vi "Read or create tokens.vi"(8 "error in":errorcluster, 10 "default value":string, 11 "key":string) -> (0 "error out":errorcluster, 3 "value":string)   [LabVIEW 2021, in "IconEditorDefaultPlugin.lvlib" / "IconEditorDefaultPlugin.lvclass"]
uses:
  <resource>/plugins/NIIconEditor/UI/Default/IconEditorDefaultPlugin.lvclass
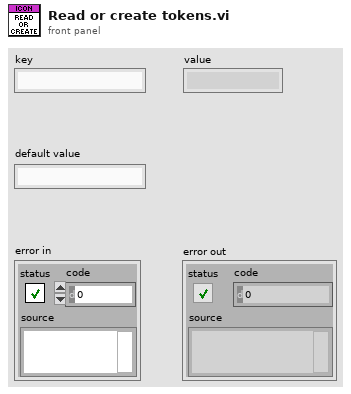
[diagram p1: front panel]
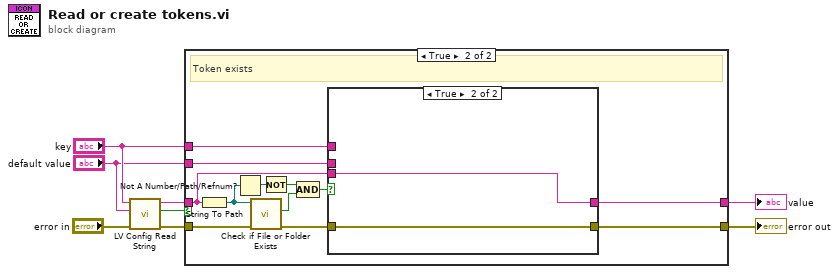
[diagram p0: block diagram]
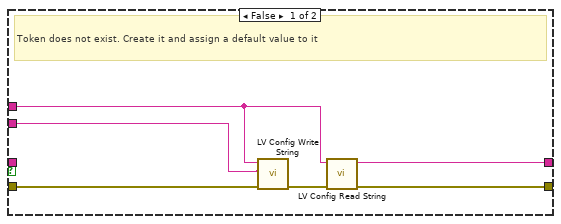
[diagram p2: hidden frame]
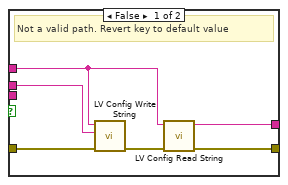
[diagram p3: hidden frame]
diagram:
  n1 = call <resource>:"LV Config Read String.vi"("error in"="error in", "default value"="default value", "key"="key") -> ("error out"=w7:errorcluster, "found?"=w6:bool, "value"=w2:string)  [unwired: 2 in]
  n2 = case shown="True" w6 {
    tunnel: w7 -> [w14 w22]
    tunnel: "key" -> [w12 w25]
    tunnel: "default value" -> [w9 w26]
    tunnel: [w11 w24] -> w4
    tunnel: [w10 w23] -> w3
    tunnel: w2 -> [_ w15]
    frame False {
      # "Token does not exist. Create it and assign a default value to it"
      n3 = call <resource>:"LV Config Write String.vi"("error in (no error)"=w14, "value"=w9, "key"=w12) -> ("error out"=w13:errorcluster)  [unwired: 4 in]
      n4 = call <resource>:"LV Config Read String.vi"("error in"=w13, "key"=w12) -> ("error out"=w11:errorcluster, "value"=w10:string)  [unwired: 3 in, 1 out]
    }
    frame True {
      # "Token exists"
      n5 = String To Path(string=w15) -> (path=w20:path)
      n6 = Not A Number/Path/Refnum?(number/path/refnum=w20) -> (NaN/Path/Refnum?=w17:bool)
      n7 = call <vilib>:"Check if File or Folder Exists.vi"("error in (no error)"=w22, "path"=w20) -> ("error out"=w21:errorcluster, "file or folder exists?"=w19:bool)  [unwired: 7 in, 1 out]
      n8 = Not(x=w17) -> (.not. x?=w16:bool)
      n9 = Compound Arithmetic op=AND(w16, w19) -> (w18:bool)
      n10 = case shown="True" w18 {
        tunnel: w21 -> [w31 w34]
        tunnel: w26 -> [w30 _]
        tunnel: w25 -> [w29 _]
        tunnel: [w28 w34] -> w24
        tunnel: [w27 w33] -> w23
        tunnel: w15 -> [_ w33]
        frame False {
          # "Not a valid path. Revert key to default value"
          n11 = call <resource>:"LV Config Write String.vi"("error in (no error)"=w31, "value"=w30, "key"=w29) -> ("error out"=w32:errorcluster)  [unwired: 4 in]
          n12 = call <resource>:"LV Config Read String.vi"("error in"=w32, "key"=w29) -> ("error out"=w28:errorcluster, "value"=w27:string)  [unwired: 3 in, 1 out]
        }
        frame True {
        }
      }
    }
  }
  "error out" <- w4
  "value" <- w3
